vi "WritePanelData_test_ringsstringscorrect.vi"(8 "error in (no error)":errorcluster, 11 "Maui.Test.DefaultDirectory in":refnum<class "Maui.Test.DefaultDirectory.lvclass">) -> (0 "error out":errorcluster, 3 "Maui.Test.DefaultDirectory out":refnum<class "Maui.Test.DefaultDirectory.lvclass">)   [LabVIEW 2020, in "Maui.Test.DefaultDirectory.lvclass"]
uses:
  Maui.Test.DefaultDirectory.lvclass
  Maui.Test.DefaultDirectory.lvclass/Maui.Test.DefaultDirectory.ctl
  <vilib>/addons/_JKI Toolkits/Caraya/classes/Assert/Assert Equal Value_Variant.vi
  <vilib>/addons/_JKI Toolkits/Caraya/classes/Test/Test.lvclass
  <vilib>/addons/_JKI Toolkits/Caraya/classes/Assert/Assert.lvclass
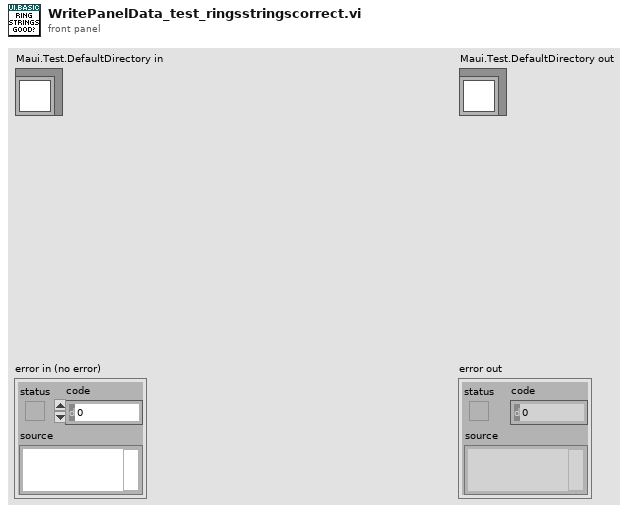
[diagram p1: front panel]
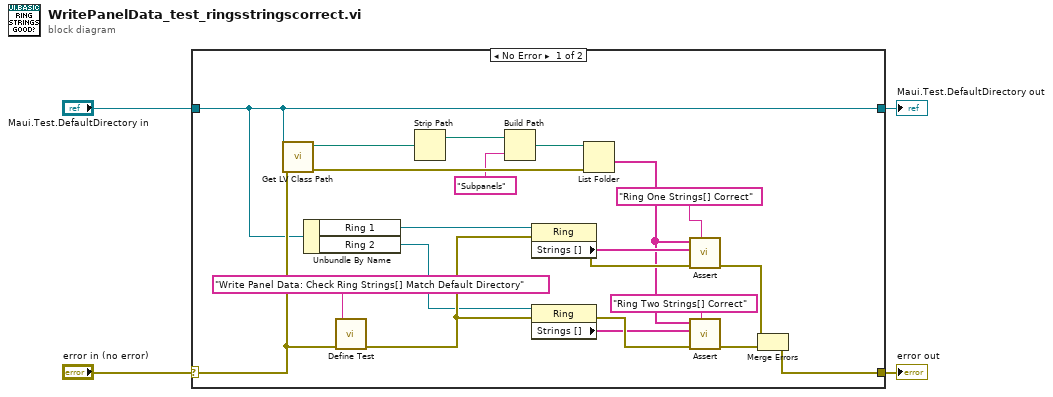
[diagram p0: block diagram]
diagram:
  n1 = case shown="No Error" "error in (no error)" {
    selector: "error in (no error)" -> [w23 w27]
    tunnel: [w22 w27] -> w3
    tunnel: [w13 w26] -> w1
    tunnel: "Maui.Test.DefaultDirectory in" -> [w13 w26]
    frame No Error {
      n2 = call <vilib>:"Get LV Class Path.vi"("error in (no error)"=w23, "object"=w13) -> ("error out"=w25:errorcluster, "class path"=w17:path)  [unwired: 8 in]
      n3 = Unbundle By Name(w13) -> ("Ring 1"=w12:refnum<vi>, "Ring 2"=w11:refnum<vi>)
      n4 = call <vilib>:"Define Test.vi"("error in (no error)"=w23, "Label (VI Title)"="Write Panel Data: Check Ring Strings[] Match Default Directory") -> ("error out"=w19:errorcluster)  [unwired: 9 in]
      n5 = Strip Path(path=w17) -> (stripped path=w16:path)  [unwired: 1 out]
      n6 = Build Path(base path=w16, name or relative path="Subpanels") -> (appended path=w14:path)
      n7 = property on="Property Node" class="Ring"(reference=w12, error in=w19) -> (error out=w20:errorcluster, "Strings []"=w7:string[])  [unwired: 1 out]
      n8 = property on="Property Node" class="Ring"(reference=w11, error in=w19) -> (error out=w18:errorcluster, "Strings []"=w9:string[])  [unwired: 1 out]
      n9 = List Folder(path=w14, error in=w25) -> (folder names=w6:string[])  [unwired: 2 in, 3 out]
      n10 = call-poly <vilib>:"Assert.vi"("Label"="Ring One Strings[] Correct" ("Label (VI Title)"), "error in (no error)"=w20, "Y"=w7, "X"=w6) -> ("error out"=w21:errorcluster)  [unwired: 7 in]
      n11 = call-poly <vilib>:"Assert.vi"("Label"="Ring Two Strings[] Correct" ("Label (VI Title)"), "error in (no error)"=w18, "Y"=w9, "X"=w6) -> ("error out"=w24:errorcluster)  [unwired: 7 in]
      n12 = Merge Errors(w21, w24) -> (w22:errorcluster)
    }
    frame Error {
    }
  }
  "error out" <- w3
  "Maui.Test.DefaultDirectory out" <- w1
